vi "Check IDs x2.vi"(8 "Addresses Cluster in":T1={"ENA1"=FALSE, "IP address 1"="172.16.14.22", "ENA2"=FALSE, "IP address 2"="172.16.14.23"}, 9 "All ID list 2":u32[](array[numeric]) format="%.0x", 10 "All ID list 1":u32[](array[numeric]) format="%.0x", 11 "LayerChipIDs":u16[](array[numeric])=[65535, 65535] format="%04x") -> (0 "Addresses Cluster out":T1={"ENA1"=FALSE, "IP address 1"="172.16.14.22", "ENA2"=FALSE, "IP address 2"="172.16.14.23"}, 2 "OK?":bool)   [LabVIEW 2015, in "VIPM2.lvlib"]
doc: "Comprova si l'adreçament és correcte.\nInclou missatge emergent si no.\nDeshabilita la FPGA no adreçada."
uses:
  VIPM2.lvlib
panel:
  out "OK2":bool
  out "OK1":bool
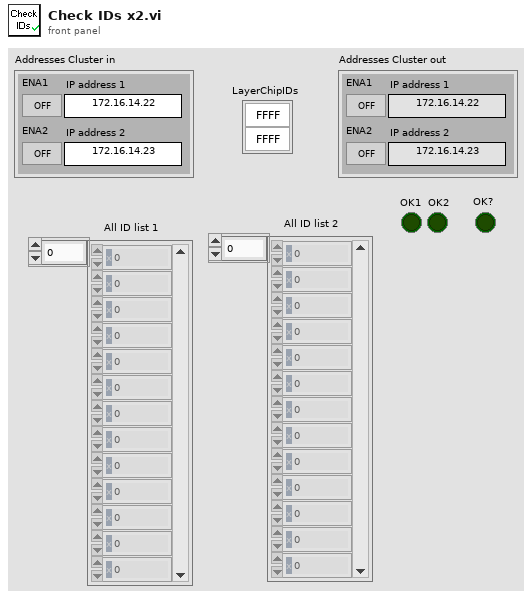
[diagram p1: front panel]
types:
  T1 = cluster{"ENA1":bool, "IP address 1":string, "ENA2":bool, "IP address 2":string}
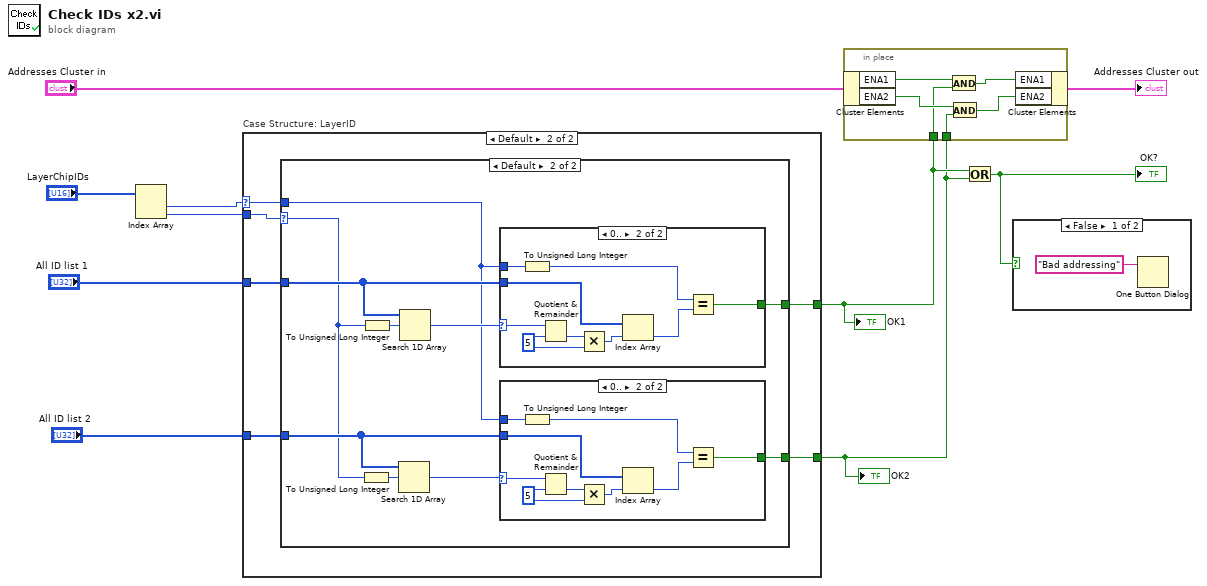
[diagram p0: block diagram]
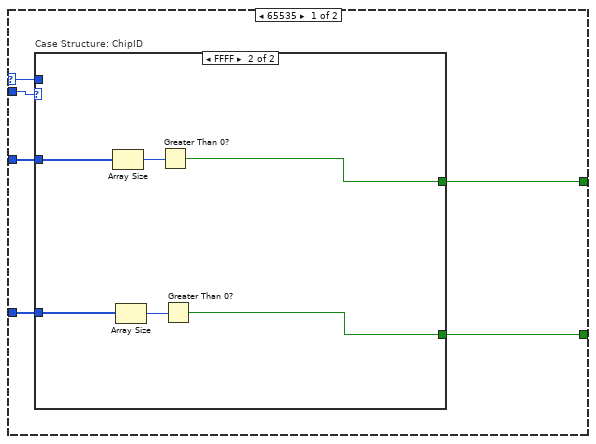
[diagram p3: hidden frame]
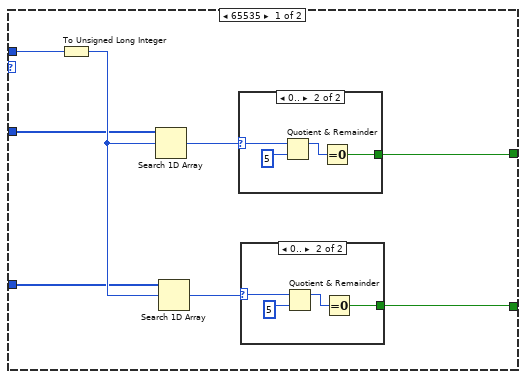
[diagram p5: hidden frame]
diagram:
  n1 = Index Array "Index Array"(array="LayerChipIDs") -> (element #1=w2:u16, element #2=w9:u16)  [unwired: 2 in]
  n2 = case "Case Structure: LayerID" shown="Default" w2 {
    selector: w2 -> [w16 w24]
    tunnel: w9 -> [w15 w23]
    tunnel: "All ID list 1" -> [w12 w28]
    tunnel: "All ID list 2" -> [w11 w27]
    tunnel: [w14 w26] -> w5
    tunnel: [w13 w25] -> w4
    frame 65535 {
      # "LayerID"
      n3 = case "Case Structure: ChipID" shown="FFFF" w15 {
        tunnel: w16 -> [_ _]
        tunnel: [_ w20] -> w14
        tunnel: [_ w17] -> w13
        tunnel: w12 -> [_ w22]
        tunnel: w11 -> [_ w18]
        frame Default {
        }
        frame 65535 {
          # "ChipID"
          n4 = Array Size(array=w22) -> (size(s)=w21:i32)
          n5 = Array Size(array=w18) -> (size(s)=w19:i32)
          n6 = Greater Than 0?(x=w21) -> (x > 0?=w20:bool)
          n7 = Greater Than 0?(x=w19) -> (x > 0?=w17:bool)
        }
      }
    }
    frame Default {
      # "LayerID"
      n8 = case shown="Default" w23 {
        selector: w23 -> [_ w45]
        tunnel: w28 -> [w32 w51]
        tunnel: w27 -> [w31 w49]
        tunnel: [w30 w48] -> w26
        tunnel: [w29 w47] -> w25
        tunnel: w24 -> [w33 w46]
        frame 65535 {
          n9 = To Unsigned Long Integer(number=w33) -> (unsigned 32bit integer=w36:u32)
          n10 = Search 1D Array(1D array=w32, element=w36) -> (index of element=w35:i32)  [unwired: 1 in]
          n11 = Search 1D Array(1D array=w31, element=w36) -> (index of element=w34:i32)  [unwired: 1 in]
          n12 = case shown="0.." w35 {
            selector: w35 -> [_ w44]
            tunnel: [_ w42] -> w30
            frame -1, Default {
            }
            frame 0.. {
              n13 = Quotient & Remainder(x=w44, y=5) -> (x-y*floor(x/y)=w41:i32)  [unwired: 1 out]
              n14 = Equal To 0?(x=w41) -> (x = 0?=w42:bool)
            }
          }
          n15 = case shown="0.." w34 {
            selector: w34 -> [_ w40]
            tunnel: [_ w38] -> w29
            frame -1, Default {
            }
            frame 0.. {
              n16 = Quotient & Remainder(x=w40, y=5) -> (x-y*floor(x/y)=w37:i32)  [unwired: 1 out]
              n17 = Equal To 0?(x=w37) -> (x = 0?=w38:bool)
            }
          }
        }
        frame Default {
          n18 = To Unsigned Long Integer(number=w45) -> (unsigned 32bit integer=w53:u32)
          n19 = To Unsigned Long Integer(number=w45) -> (unsigned 32bit integer=w54:u32)
          n20 = Search 1D Array(1D array=w49, element=w53) -> (index of element=w50:i32)  [unwired: 1 in]
          n21 = Search 1D Array(1D array=w51, element=w54) -> (index of element=w52:i32)  [unwired: 1 in]
          n22 = case shown="0.." w52 {
            selector: w52 -> [_ w72]
            tunnel: w51 -> [_ w71]
            tunnel: w46 -> [_ w70]
            tunnel: [_ w67] -> w48
            frame -1, Default {
            }
            frame 0.. {
              w65 = 5 ("y")
              n23 = To Unsigned Long Integer(number=w70) -> (unsigned 32bit integer=w69:u32)
              n24 = Quotient & Remainder(x=w72, y=w65) -> (floor(x/y)=w66:i32)  [unwired: 1 out]
              n25 = Multiply(x=w66, y=w65) -> (x*y=w64:i32)
              n26 = Index Array "Index Array"(array=w71, index=w64) -> (element=w68:u32)
              n27 = Equal?(x=w69, y=w68) -> (x = y?=w67:bool)
            }
          }
          n28 = case shown="0.." w50 {
            selector: w50 -> [_ w63]
            tunnel: w49 -> [_ w62]
            tunnel: w46 -> [_ w61]
            tunnel: [_ w58] -> w47
            frame -1, Default {
            }
            frame 0.. {
              w55 = 5 ("y")
              n29 = To Unsigned Long Integer(number=w61) -> (unsigned 32bit integer=w60:u32)
              n30 = Quotient & Remainder(x=w63, y=w55) -> (floor(x/y)=w56:i32)  [unwired: 1 out]
              n31 = Multiply(x=w56, y=w55) -> (x*y=w57:i32)
              n32 = Index Array "Index Array"(array=w62, index=w57) -> (element=w59:u32)
              n33 = Equal?(x=w60, y=w59) -> (x = y?=w58:bool)
            }
          }
        }
      }
    }
  }
  "OK1" <- w5
  "OK2" <- w4
  n34 = in-place "In Place Element Structure" {
    in-place-border: w5 -> [w74]
    in-place-border: w4 -> [w73]
    n35 = in-place-cluster #1("Addresses Cluster in") -> ("ENA1"=w78:bool, "ENA2"=w77:bool)
    n36 = And(x=w78, y=w74) -> (x .and. y?=w76:bool)
    n37 = And(x=w77, y=w73) -> (x .and. y?=w75:bool)
    n38 = in-place-cluster #1("ENA1"=w76, "ENA2"=w75) -> (→"Addresses Cluster out":T1)
  }
  n39 = Or(x=w5, y=w4) -> (x .or. y?=w1:bool)
  "OK?" <- w1
  n40 = case shown="False" w1 {
    frame False {
      n41 = One Button Dialog(message="Bad addressing") -> ()  [unwired: 1 in, 1 out]
    }
    frame True {
    }
  }
